vi "AcquireSet.vi"(7 "参数查询(0)/设置(1)":bool, 8 "error in (no error)":errorcluster caption="错误输入（无错误）", 9 "设置参数":string, 10 "ACQUIRE命令子系统":string(combo), 11 "VISA资源名称":refnum<visa-resource-name>) -> (0 "error out":errorcluster caption="错误输出", 1 "查询返回字节数":u32, 2 "查询返回":string, 3 "VISA资源名称 2":refnum<visa-resource-name>)   [LabVIEW 2018]
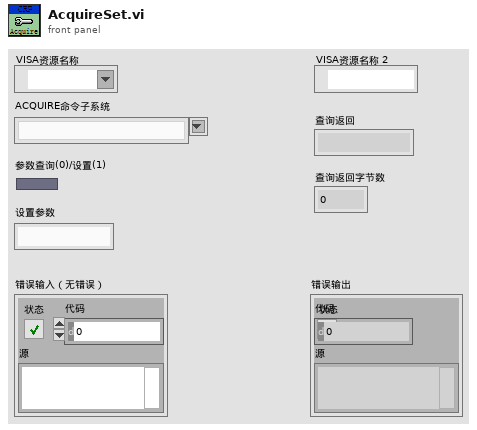
[diagram p1: front panel]
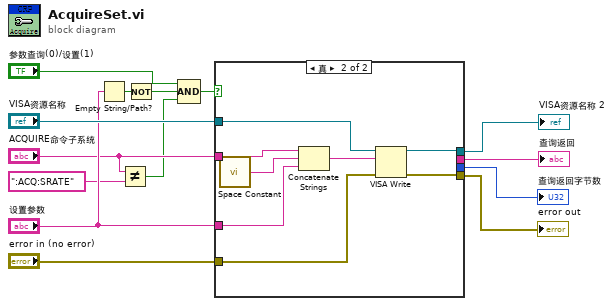
[diagram p0: block diagram]
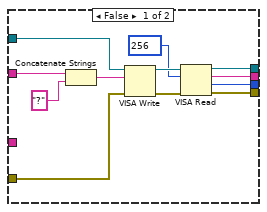
[diagram p2: hidden frame]
diagram:
  n1 = Empty String/Path?(string/path="设置参数") -> (empty?=w7:bool)
  n2 = Not Equal?(x="ACQUIRE命令子系统", y=":ACQ:SRATE") -> (x != y?=w1:bool)
  n3 = Not(x=w7) -> (.not. x?=w4:bool)
  n4 = Compound Arithmetic op=AND ("复合运算")("参数查询(0)/设置(1)", w4, w1) -> (w9:bool)
  n5 = case shown="真" w9 {
    tunnel: "设置参数" -> [_ w33]
    tunnel: "error in (no error)" -> [w16 w28]
    tunnel: [w22 w30] -> w13
    tunnel: [w21 _] -> w6
    tunnel: [w20 w31] -> w12
    tunnel: "ACQUIRE命令子系统" -> [w19 w32]
    tunnel: "VISA资源名称" -> [w17 w27]
    tunnel: [w15 _] -> w5
    frame False {
      n6 = Concatenate Strings(w19, "?") -> (w26:string)
      n7 = VISA Write(VISA resource name=w17, write buffer=w26, error in (no error)=w16) -> (VISA resource name out=w24:refnum<visa-resource-name>, error out=w25:errorcluster)  [unwired: 1 out]
      n8 = VISA Read(VISA resource name=w24, byte count=u32 256 ("字节总数"), error in (no error)=w25) -> (VISA resource name out=w20:refnum<visa-resource-name>, read buffer=w21:string, return count=w15:u32, error out=w22:errorcluster)
    }
    frame True {
      n9 = call <vilib>:"Space Constant.vi"() -> ("String"=w34:string)
      n10 = Concatenate Strings(w32, w34, w33) -> (w29:string)
      n11 = VISA Write(VISA resource name=w27, write buffer=w29, error in (no error)=w28) -> (VISA resource name out=w31:refnum<visa-resource-name>, error out=w30:errorcluster)  [unwired: 1 out]
    }
  }
  "error out" <- w13
  "VISA资源名称 2" <- w12
  "查询返回" <- w6
  "查询返回字节数" <- w5
